vi "Adam_Ch_on_off.vi"(1 "Ch State":T1, 2 "ADAM Ch Names":string[](array[string])=["EnFlo Tun:Ultrasonic:Fixed"]) -> ()   [LabVIEW 2010]
uses:
  ADAM Controls/Channel_State.ctl
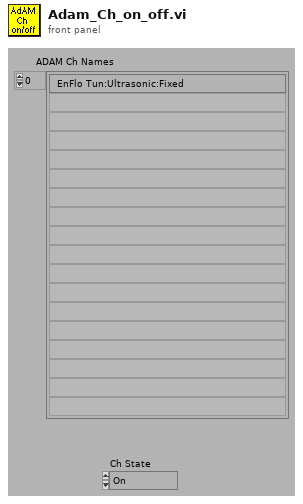
[diagram p1: front panel]
types:
  T1 = typedef "Channel_State.ctl" = enum16{"On", "Off", "Always On", "Always Off"}
  T2 = typedef "Ch_description_ADAM.ctl" = cluster{"Ch Name":string, "Type":T3, "Function":T4, "Ch State":T1, "Calibration type":T5, "A":dbl, "B":dbl, "C":dbl, "D":dbl, "Comments":string, "Address":T6, "String":string, "Duty":u16}
  T3 = typedef "Module_type_ADAM.ctl" = enum16{"4011", "4012", "4013", "4014", "4016", "4017", "4018", "4021", "4050", "4052", "4053", "4060", "4080", "5000", "5017", "5018", "5024", "5051", "5056", "5060", "6060", "Tracker", "WEST", "GILL", "JEM", "VICI", "Vaisala", "DRUCK", "Run VI Named:", "IR2100", "PPT", "Comparator", "VIRTUAL", "Hold Value", "Read A", "Read Ch", "Coded", "Client Info", "Web Client", "X10", "Test"}
  T4 = typedef "Function_ADAM.ctl" = enum16{"Analogue Input", "Digital Input", "Event counter", "Event rate", "Analogue Output", "Digital Output", "Relay Output"}
  T5 = typedef "Calib_type_ADAM.ctl" = enum16{"Raw", "Bx + A", "Cx^2 + Bx + A", "Dx^3 + Cx^2 + Bx + A", "In Band", "Hi-Tec Q", "Hi-Tec M_dot", "Text"}
  T6 = typedef "Address.ctl" = cluster{"Main":i32, "Ch.":i32, "Sub":i32, "Port Name":string}
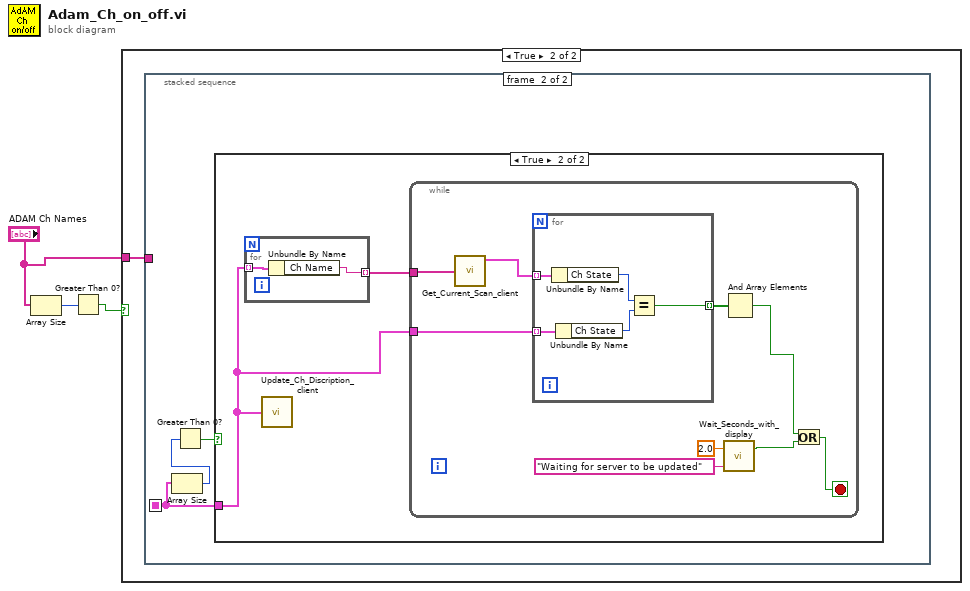
[diagram p0: block diagram]
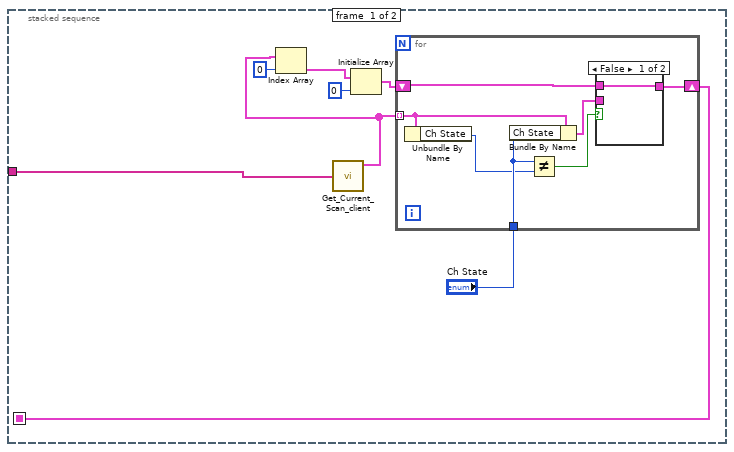
[diagram p3: hidden frame]
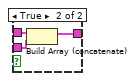
[diagram p4: hidden frame]
diagram:
  n1 = Array Size(array="ADAM Ch Names") -> (size(s)=w3:i32)
  n2 = Greater Than 0?(x=w3) -> (x > 0?=w2:bool)
  n3 = case shown="True" w2 {
    tunnel: "ADAM Ch Names" -> [_ w4]
    frame False {
    }
    frame True {
      n4 = stacked-sequence {
        seq-local: [w7 _] -> [_ w26]
        tunnel: w4 -> [w6 _]
        frame #0 {
          n5 = call "Get_Current_Scan_client.vi"("ADAM Ch Names"=w6) -> ("Ch Description Array"=w9:T2[])  [unwired: 3 out]
          n6 = Index Array(array=w9, index=0) -> (element=w8:T2)
          n7 = Initialize Array(w8, 0 ("dimension size")) -> (w12:T2[])
          n8 = for {
            tunnel: w9 -> [w19] mode=indexing
            shift-right: [w16] -> w7
            shift-left: w12 -> [w17]
            tunnel: "Ch State" -> [w18]
            n9 = Unbundle By Name(w19) -> ("Ch State"=w15:T1)
            n10 = Bundle By Name(cluster=w19, "Ch State"=w18) -> (w14:T2)
            n11 = Not Equal?(x=w18, y=w15) -> (x != y?=w13:bool)
            n12 = case shown="False" w13 {
              tunnel: w17 -> [w20 w23]
              tunnel: w14 -> [_ w22]
              tunnel: [w20 w21] -> w16
              frame False {
              }
              frame True {
                n13 = Build Array (concatenate)(w23, w22) -> (w21:T2[])
              }
            }
          }
        }
        frame #1 {
          n14 = Array Size(array=w26) -> (size(s)=w25:i32)
          n15 = Greater Than 0?(x=w25) -> (x > 0?=w24:bool)
          n16 = case shown="True" w24 {
            tunnel: w26 -> [_ w27]
            frame False {
            }
            frame True {
              n17 = for {
                tunnel: w27 -> [w44] mode=indexing
                tunnel: [w43] -> w28 mode=indexing
                n18 = Unbundle By Name(w44) -> ("Ch Name"=w43:string)
              }
              n19 = call "Update_Ch_Discription_client.vi"("Channels to update In"=w27) -> ()  [unwired: 1 out]
              n20 = while {
                tunnel: w28 -> [w37]
                tunnel: w27 -> [w35]
                stop <- w31 stop-if-true
                n21 = call "Get_Current_Scan_client.vi"("ADAM Ch Names"=w37) -> ("Ch Description Array"=w36:T2[])  [unwired: 3 out]
                n22 = for {
                  tunnel: w36 -> [w42] mode=indexing
                  tunnel: w35 -> [w41] mode=indexing
                  tunnel: [w38] -> w34 mode=indexing
                  n23 = Unbundle By Name(w42) -> ("Ch State"=w39:T1)
                  n24 = Unbundle By Name(w41) -> ("Ch State"=w40:T1)
                  n25 = Equal?(x=w39, y=w40) -> (x = y?=w38:bool)
                }
                n26 = call "Wait_Seconds_with_display.vi"("Message"="Waiting for server to be updated", "Seconds to wait"=2.0) -> ("Stopped"=w32:bool)  [unwired: 1 out]
                n27 = And Array Elements(Boolean array=w34) -> (logical AND=w33:bool)
                n28 = Or(x=w33, y=w32) -> (x .or. y?=w31:bool)
              }
            }
          }
        }
      }
    }
  }
